vi "registerWindowCloseCallback.vi"(8 "error in (no error)":errorcluster, 11 "Actor wUI in":refnum<class "Actor wUI.lvclass">) -> (0 "error out":errorcluster, 3 "Actor wUI out":refnum<class "Actor wUI.lvclass">)   [LabVIEW 2017, in "Framework.lvlib" / "Actor wUI.lvclass"]
uses:
  Actor wUI.lvclass
  Actor wUI.lvclass/Actor wUI.ctl
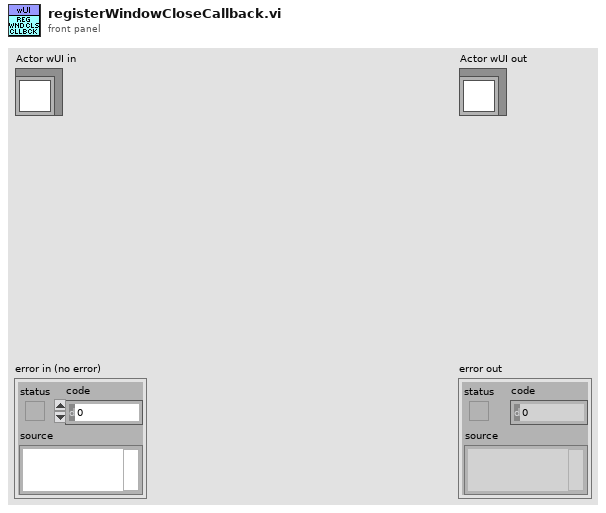
[diagram p1: front panel]
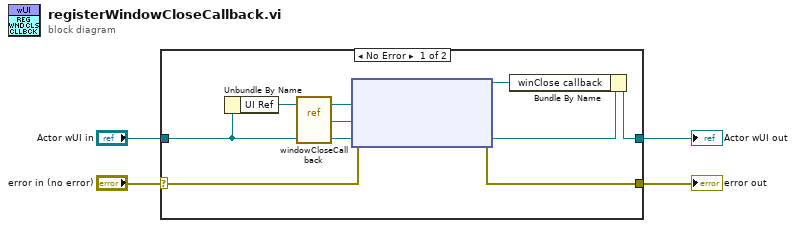
[diagram p0: block diagram]
diagram:
  n1 = case shown="No Error" "error in (no error)" {
    selector: "error in (no error)" -> [w8 w13]
    tunnel: [w7 w13] -> w3
    tunnel: [w6 w12] -> w1
    tunnel: "Actor wUI in" -> [w9 w12]
    frame No Error {
      n2 = Unbundle By Name(w9) -> ("UI Ref"=w11:refnum<vi>)
      n3 = vi-ref "windowCloseCallback.vi"() -> ("vi reference"=w10:refnum<vi>)
      n4 = node(w8, w11, w10, w9) -> (w5:refnum<k27>, w7:errorcluster)  [unwired: 1 in]
      n5 = Bundle By Name(cluster=w9, "winClose callback"=w5) -> (w6:refnum<class "Actor wUI.lvclass">)
    }
    frame Error {
    }
  }
  "error out" <- w3
  "Actor wUI out" <- w1
